vi "Open FP in SP.vi"(8 "error in (no error)":errorcluster, 11 "Monedas in":refnum<class "Monedas.lvclass">) -> (0 "error out":errorcluster, 3 "Monedas out":refnum<class "Monedas.lvclass">)   [LabVIEW 2020, in "Monedas.lvlib" / "Monedas.lvclass"]
uses:
  Monedas.lvclass
  Monedas.lvclass/Monedas.ctl
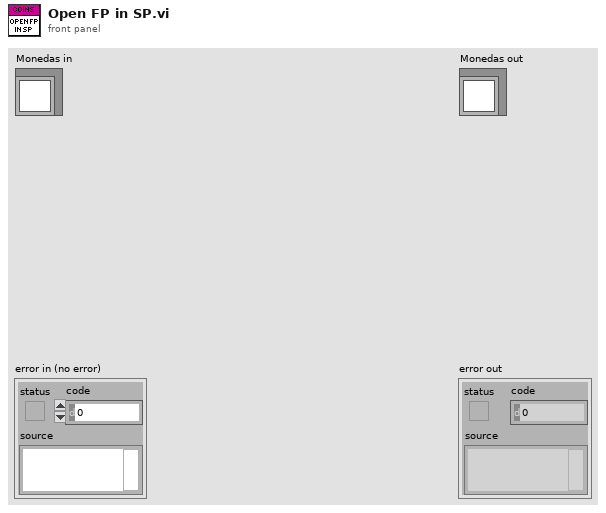
[diagram p1: front panel]
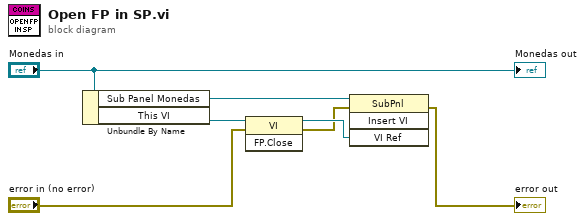
[diagram p0: block diagram]
diagram:
  n1 = Unbundle By Name("Monedas in") -> ("Sub Panel Monedas"=w6:refnum<vi>, "This VI"=w5:refnum<vi>)
  n2 = invoke class="VI" method="FP.Close"(reference=w5, error in="error in (no error)") -> (reference out=w4:refnum<vi>, error out=w2:errorcluster)  [unwired: 1 in, 1 out]
  n3 = invoke class="SubPnl" method="Insert VI"(reference=w6, error in=w2, "VI Ref"=w4) -> (error out=→"error out":errorcluster)  [unwired: 1 in, 3 out]
  "Monedas out" <- "Monedas in"
